vi "heating_visu check.vi"() -> ()   [LabVIEW 2019]
uses:
  Heating.lvlib
  ctl/ZY_state_short.ctl
  ctl/Z.ctl
  ctl/Y_source.ctl
  ctl/Z_State.ctl
  ctl/ZM_State.ctl
  ctl/Y_short.ctl
  ctl/Y_state.ctl
  Inputs/Ctl/Parameter State short.ctl
  Alarms/Ctl/ALR_Status_short.ctl
  ctl/ZY_control.ctl
  Inputs/Inputs.lvlib
  Alarms/Alarms.lvlib
  Reg/ctl/Z_State.ctl
  Reg/control.lvlib
  Reg/ctl/Y_state.ctl
panel:
  out "Write Enable 2":bool
  out "Write Enable":bool
  out "HT1_out":T1 {"Y"."SP" step=0.01 format="%.2f"; "Y"."Y" format="%.2f"; "Y"."PV" step=0.01 format="%.2f"; "Y"."SP_Set" step=0.01 format="%.2f"}
  out "ZY_out 2":T10={"Z_HSw"=1, "Z_HSetState"=enum."on", "Y_HSw"=1, "Y_HSetState"=enum."auto", "SP"=0.0, "Y_H"=0.0, "Reset_ALR"=FALSE} {"Y_H" step=1.0; "SP" step=0.01 format="%.2f"}
  out "ZY_out":T10={"Z_HSw"=1, "Z_HSetState"=enum."on", "Y_HSw"=1, "Y_HSetState"=enum."auto", "SP"=0.0, "Y_H"=0.0, "Reset_ALR"=FALSE} {"Y_H" step=1.0; "SP" step=0.01 format="%.2f"}
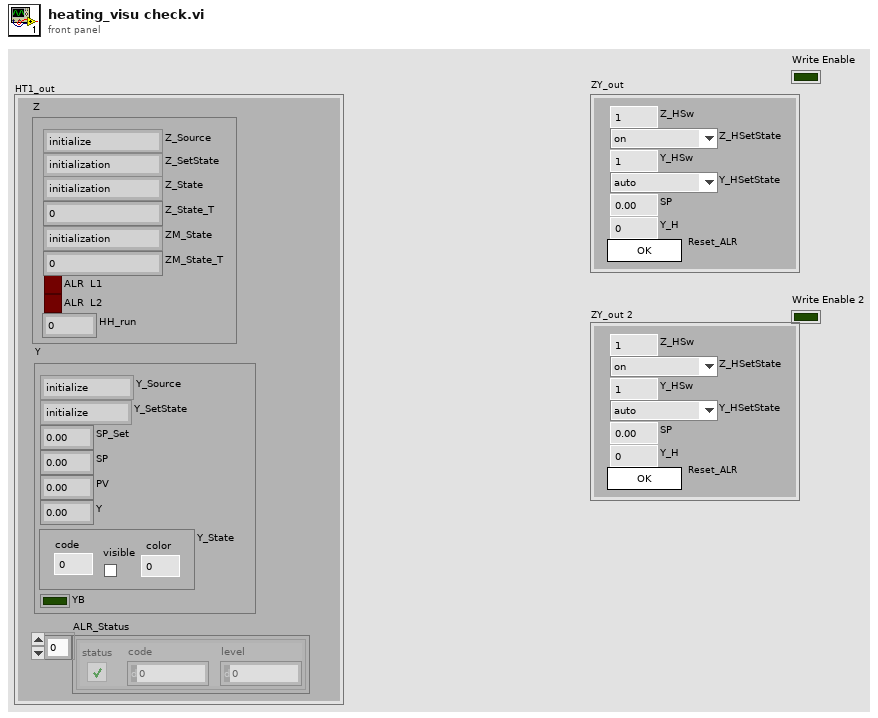
[diagram p1: front panel]
types:
  T1 = typedef "Heating.lvlib/ZY_state_short.ctl" = cluster{"Z":T2, "Y":T6, "ALR_Status":T9[]}
  T2 = typedef "Heating.lvlib/Z.ctl" = cluster{"Z_Source":T3, "Z_SetState":T4, "Z_State":T4, "Z_State_T":u32, "ZM_State":T5, "ZM_State_T":u32, "ALR  L1":bool, "ALR  L2":bool, "HH_run":i32}
  T3 = typedef "Heating.lvlib/Y_source.ctl" = enum8{"initialize", "local disabled", "local hand", "hand", "auto", "dist"}
  T4 = typedef "Heating.lvlib/Z_State.ctl" = enum8{"initialization", "alarm", "disabled", "not ready", "stop ready", "reserv", "switched off", "reserv2", "switched on", "check", "on min", "decrease out", "on", "increase out", "on max"}
  T5 = typedef "Heating.lvlib/ZM_State.ctl" = enum8{"initialization", "stop", "start_cmd", "contactor_on_cmd", "heating", "on", "stop_cmd", "power_down", "contactor_off_cmd", "cooling", "restart_delay"}
  T6 = typedef "Heating.lvlib/Y_short.ctl" = cluster{"Y_Source":T3, "Y_SetState":T7, "SP_Set":dbl, "SP":dbl, "PV":dbl, "Y":dbl, "Y_State":T8, "YB":bool}
  T7 = typedef "Heating.lvlib/Y_state.ctl" = enum8{"initialize", "alarm", "min", "stop", "hand", "auto", "max"}
  T8 = typedef "Inputs.lvlib/Parameter State short.ctl" = cluster{"code":i32, "visible":bool, "color":u32}
  T9 = typedef "Alarms.lvlib/ALR_Status_short.ctl" = cluster{"status":bool, "code":i32, "level":i32}
  T10 = typedef "Heating.lvlib/ZY_control.ctl" = cluster{"Z_HSw":u32, "Z_HSetState":T11, "Y_HSw":u32, "Y_HSetState":T12, "SP":dbl, "Y_H":dbl, "Reset_ALR":bool}
  T11 = typedef "control.lvlib/Z_State.ctl" = enum8{"initialization", "alarm", "disabled", "not ready", "stop ready", "reserv", "switched off", "reserv2", "switched on", "check", "on min", "decrease out", "on", "increase out", "on max"}
  T12 = typedef "control.lvlib/Y_state.ctl" = enum8{"initialize", "alarm", "min", "stop", "hand", "auto", "max"}
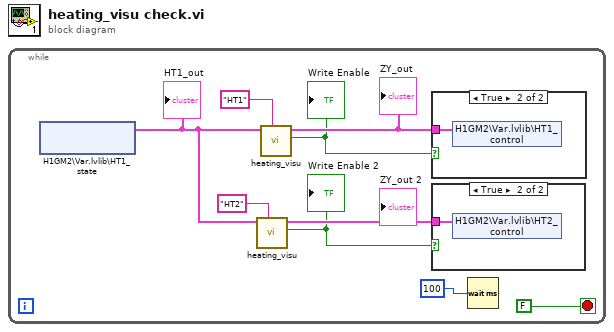
[diagram p0: block diagram]
diagram:
  n1 = while {
    stop <- FALSE stop-if-true
    n2 = shared-variable "H1GM2\\Var.lvlib\\HT1_state"() -> (w1:T1)  [unwired: 2 in, 2 out]
    "HT1_out" <- w1
    n3 = call "heating_visu.vi"("name"="HT2", "ZY_In"=w1) -> ("Write Enable"=w3:bool, "ZY_out"=w5:T10)  [unwired: 7 in, 1 out]
    "ZY_out 2" <- w5
    "Write Enable 2" <- w3
    n4 = call "heating_visu.vi"("name"="HT1", "ZY_In"=w1) -> ("Write Enable"=w4:bool, "ZY_out"=w6:T10)  [unwired: 7 in, 1 out]
    "ZY_out" <- w6
    "Write Enable" <- w4
    n5 = case shown="True" w4 {
      tunnel: w6 -> [_ w11]
      frame False {
      }
      frame True {
        n6 = shared-variable "H1GM2\\Var.lvlib\\HT1_control"(w11) -> ()  [unwired: 1 in, 1 out]
      }
    }
    n7 = case shown="True" w3 {
      tunnel: w5 -> [_ w10]
      frame False {
      }
      frame True {
        n8 = shared-variable "H1GM2\\Var.lvlib\\HT2_control"(w10) -> ()  [unwired: 1 in, 1 out]
      }
    }
    n9 = Wait (ms)(milliseconds to wait=u32 100) -> ()  [unwired: 1 out]
  }
